vi "AutoTurn.vi"(8 "error in (no error)":errorcluster, 9 "TimeOut (s)":dbl, 10 "MaxSpeed (ft/s)":dbl, 11 "degrees":dbl) -> (0 "error out":errorcluster)   [LabVIEW 2020]
doc: "Turn for auto\ninputs:\n--Timer\n-error in\n\noutputs:\n--error out"
uses:
  <vilib>/Utility/semaphor.llb/Obtain Semaphore Reference.vi
  <vilib>/Rock Robotics/WPI/ThirdParty/JAS_Junk/TrajLib/Timer_Reset.vi
  <vilib>/Rock Robotics/WPI/ThirdParty/JAS_Junk/TrajLib/Trajectory_Library.lvlib
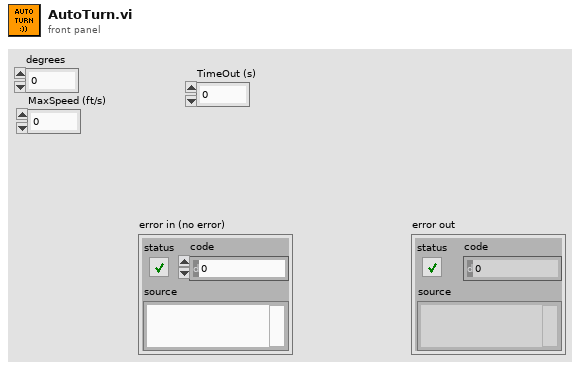
[diagram p1: front panel]
types:
  T1 = typedef "Trajectory_Library.lvlib/TIMER.ctl" = cluster{"StartTime":dbl, "Accumulated TIme":dbl, "Running":bool, "semaphore":T2}
  T2 = typedef "Semaphore RefNum" = refnum<k1>
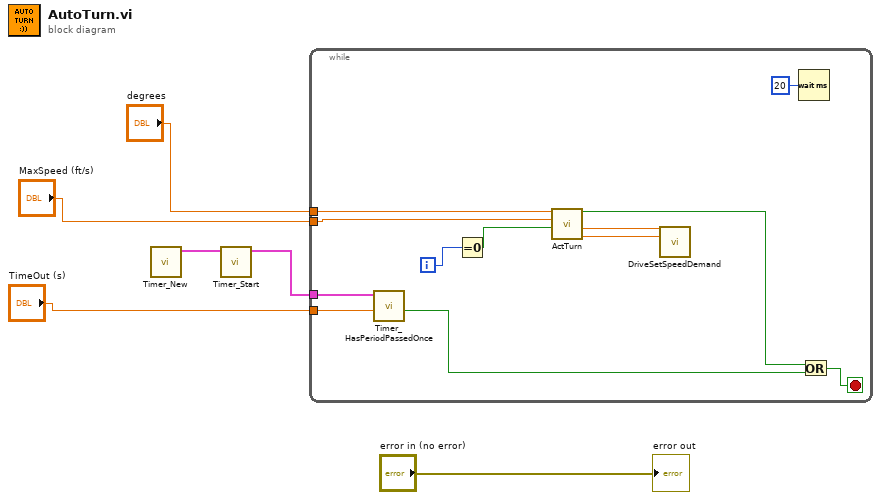
[diagram p0: block diagram]
diagram:
  n1 = call <vilib>:"Timer_New.vi"() -> ("TIMER"=w3:T1)  [unwired: 11 in]
  n2 = call <vilib>:"Timer_Start.vi"("in Timer"=w3) -> ("out Timer"=w2:T1)  [unwired: 10 in]
  n3 = while {
    tunnel: "degrees" -> [w12]
    tunnel: "MaxSpeed (ft/s)" -> [w11]
    tunnel: w2 -> [w17]
    tunnel: "TimeOut (s)" -> [w16]
    i -> [w18]
    stop <- w14 stop-if-true
    n4 = call <vilib>:"Timer_HasPeriodPassedOnce.vi"("Period"=w16, "in Timer"=w17) -> ("Expired"=w15:bool)  [unwired: 7 in, 2 out]
    n5 = Equal To 0?(x=w18) -> (x = 0?=w10:bool)
    n6 = call "ActTurn.vi"("FirstTime"=w10, "MaxSpeed (ft/s)"=w11, "Degrees"=w12) -> ("RightSpeedDemand"=w8:dbl, "LeftSpeedDemand"=w7:dbl, "Done"=w9:bool)  [unwired: 5 in, 1 out]
    n7 = call "DriveSetSpeedDemand.vi"("RSpeedDemand (ft/s)"=w8, "LSpeedDemand (ft/s)"=w7) -> ()  [unwired: 10 in]
    n8 = Wait (ms)(milliseconds to wait=u32 20) -> ()  [unwired: 1 out]
    n9 = Or(x=w9, y=w15) -> (x .or. y?=w14:bool)
  }
  "error out" <- "error in (no error)"
